vi "Place a dot on each strip and center.vi"(10 "Clamp Points (Max Clamp 1)":T1, 11 "Image":T2) -> (3 "Image Out":T2)   [LabVIEW 2018]
uses:
  <vilib>/vision/Image Controls.llb/IMAQ Image.ctl
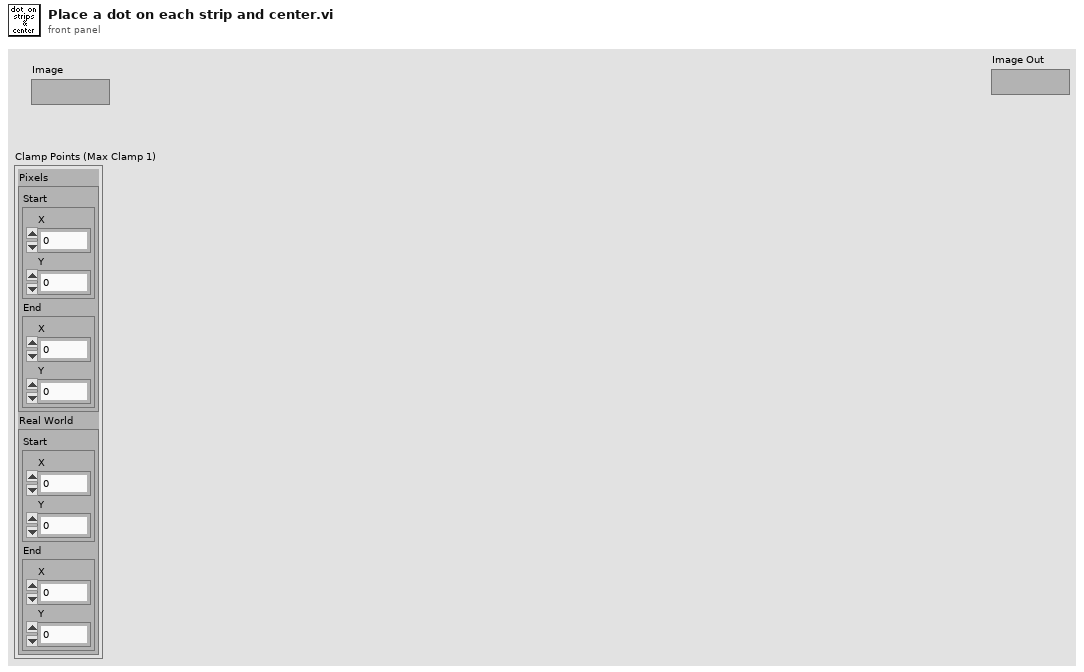
[diagram p1: front panel]
types:
  T1 = cluster{"Pixels ":cluster{"Start":cluster{"X":dbl, "Y":dbl}, "End":cluster{"X":dbl, "Y":dbl}}, "Real World":cluster{"Start":cluster{"X":dbl, "Y":dbl}, "End":cluster{"X":dbl, "Y":dbl}}}
  T2 = typedef "IMAQ Image.ctl" = refnum<image>
  T3 = cluster{"Start":cluster{"X":dbl, "Y":dbl}, "End":cluster{"X":dbl, "Y":dbl}}
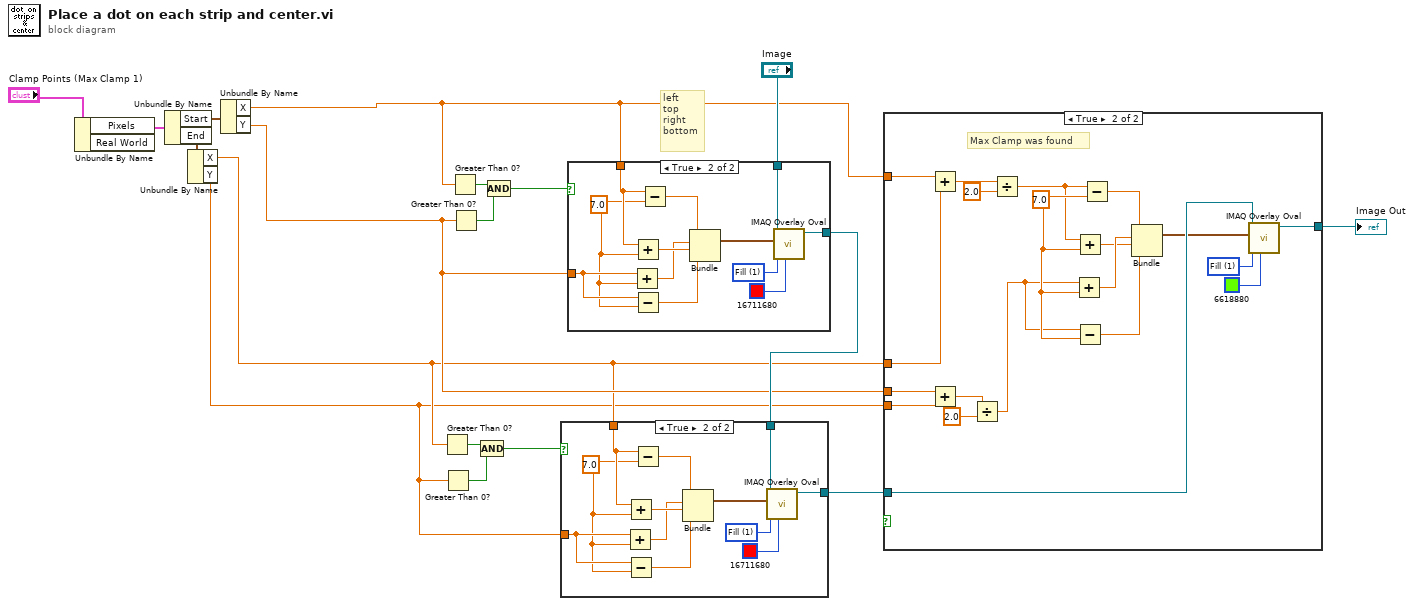
[diagram p0: block diagram]
diagram:
  # "left\ntop\nright\nbottom"
  n1 = Unbundle By Name("Clamp Points (Max Clamp 1)") -> ("Pixels"=w10:T3)  [unwired: 1 out]
  n2 = Unbundle By Name(w10) -> ("Start"=w9:cluster{"X":dbl, "Y":dbl}, "End"=w8:cluster{"X":dbl, "Y":dbl})
  n3 = Unbundle By Name(w8) -> ("X"=w3:dbl, "Y"=w2:dbl)
  n4 = Unbundle By Name(w9) -> ("X"=w1:dbl, "Y"=w4:dbl)
  n5 = Greater Than 0?(x=w3) -> (x > 0?=w14:bool)
  n6 = Greater Than 0?(x=w2) -> (x > 0?=w15:bool)
  n7 = Greater Than 0?(x=w1) -> (x > 0?=w18:bool)
  n8 = Greater Than 0?(x=w4) -> (x > 0?=w17:bool)
  n9 = Compound Arithmetic op=AND(w14, w15) -> (w6:bool)
  n10 = Compound Arithmetic op=AND(w18, w17) -> (w5:bool)
  n11 = case shown="True" w5 {
    tunnel: w1 -> [_ w25]
    tunnel: "Image" -> [w19 w28]
    tunnel: [w19 w27] -> w13
    tunnel: w4 -> [_ w22]
    frame False {
    }
    frame True {
      w30 = u32 1 items=["Frame", "Fill"] ("Drawing Mode (Frame)")
      w21 = 7.0 ("y")
      n12 = Add(x=w22, y=w21) -> (x+y=w23:dbl)
      n13 = Add(x=w25, y=w21) -> (x+y=w24:dbl)
      n14 = Subtract(x=w22, y=w21) -> (x-y=w20:dbl)
      n15 = Subtract(x=w25, y=w21) -> (x-y=w26:dbl)
      n16 = Bundle(w26, w23, w24, w20) -> (w31:cluster{dbl, dbl, dbl, dbl})  [unwired: 1 in]
      n17 = call "IMAQ Overlay Oval"("Color"=u32 16711680, "Drawing Mode (Frame)"=w30, "Bounding Rectangle"=w31, "Image"=w28) -> ("Image Out"=w27:T2)  [unwired: 6 in, 1 out]
    }
  }
  n18 = case shown="True" w6 {
    tunnel: w3 -> [_ w38]
    tunnel: w13 -> [w32 w41]
    tunnel: [w32 w40] -> w12
    tunnel: w2 -> [_ w35]
    frame False {
    }
    frame True {
      w43 = u32 1 items=["Frame", "Fill"] ("Drawing Mode (Frame)")
      w34 = 7.0 ("y")
      n19 = Add(x=w35, y=w34) -> (x+y=w36:dbl)
      n20 = Add(x=w38, y=w34) -> (x+y=w37:dbl)
      n21 = Subtract(x=w35, y=w34) -> (x-y=w33:dbl)
      n22 = Subtract(x=w38, y=w34) -> (x-y=w39:dbl)
      n23 = Bundle(w39, w36, w37, w33) -> (w44:cluster{dbl, dbl, dbl, dbl})  [unwired: 1 in]
      n24 = call "IMAQ Overlay Oval"("Color"=u32 16711680, "Drawing Mode (Frame)"=w43, "Bounding Rectangle"=w44, "Image"=w41) -> ("Image Out"=w40:T2)  [unwired: 6 in, 1 out]
    }
  }
  n25 = case shown="True" {
    selector: _ -> [_ _]
    tunnel: w3 -> [_ w65]
    tunnel: w4 -> [_ w56]
    tunnel: w2 -> [_ w55]
    tunnel: w12 -> [w45 w49]
    tunnel: [w45 w47] -> w11
    tunnel: w1 -> [_ w46]
    frame False {
      # "Max Clamp wasn't found"
    }
    frame True {
      w50 = u32 1 items=["Frame", "Fill"] ("Drawing Mode (Frame)")
      w63 = 7.0 ("y")
      # "Max Clamp was found"
      n26 = Add(x=w46, y=w65) -> (x+y=w59:dbl)
      n27 = Add(x=w56, y=w55) -> (x+y=w53:dbl)
      n28 = Divide(x=w53, y=2.0) -> (x/y=w52:dbl)
      n29 = Divide(x=w59, y=2.0) -> (x/y=w57:dbl)
      n30 = Add(x=w52, y=w63) -> (x+y=w62:dbl)
      n31 = Add(x=w57, y=w63) -> (x+y=w61:dbl)
      n32 = Subtract(x=w52, y=w63) -> (x-y=w64:dbl)
      n33 = Subtract(x=w57, y=w63) -> (x-y=w60:dbl)
      n34 = Bundle(w60, w62, w61, w64) -> (w48:cluster{dbl, dbl, dbl, dbl})  [unwired: 1 in]
      n35 = call "IMAQ Overlay Oval"("Color"=u32 6618880, "Drawing Mode (Frame)"=w50, "Bounding Rectangle"=w48, "Image"=w49) -> ("Image Out"=w47:T2)  [unwired: 6 in, 1 out]
    }
  }
  "Image Out" <- w11
